vi "SQL查询.vi"(7 "condition":string, 8 "error in (no error)":errorcluster, 9 "columns":string[](array[string]), 10 "table输入":string(combo), 11 "database":string(combo)) -> (0 "error out":errorcluster, 1 "拆分数据":bool, 2 "columns输出":string[](array[string]), 3 "data":string[][](table))   [LabVIEW 2016, in "数据传输系统-02.lvlib"]
uses:
  <vilib>/Utility/sysdir.llb/System Directory Type.ctl
  <vilib>/addons/database/Connection.llb/DB Tools Open Connec (String).vi
  <vilib>/addons/database/_DB Variant To Data/Database Variant To Data.xnode
  <vilib>/addons/database/NI_Database_API.lvlib
panel:
  out "error out 2":errorcluster
  out "结果字符串":string
  out "元素":string
  out "子数组":string[](array[string])
  # "时间 > #2021/01/15 08:00:00#and 时间 < #2021/04/15 08:00:00# order by 时间 asc"
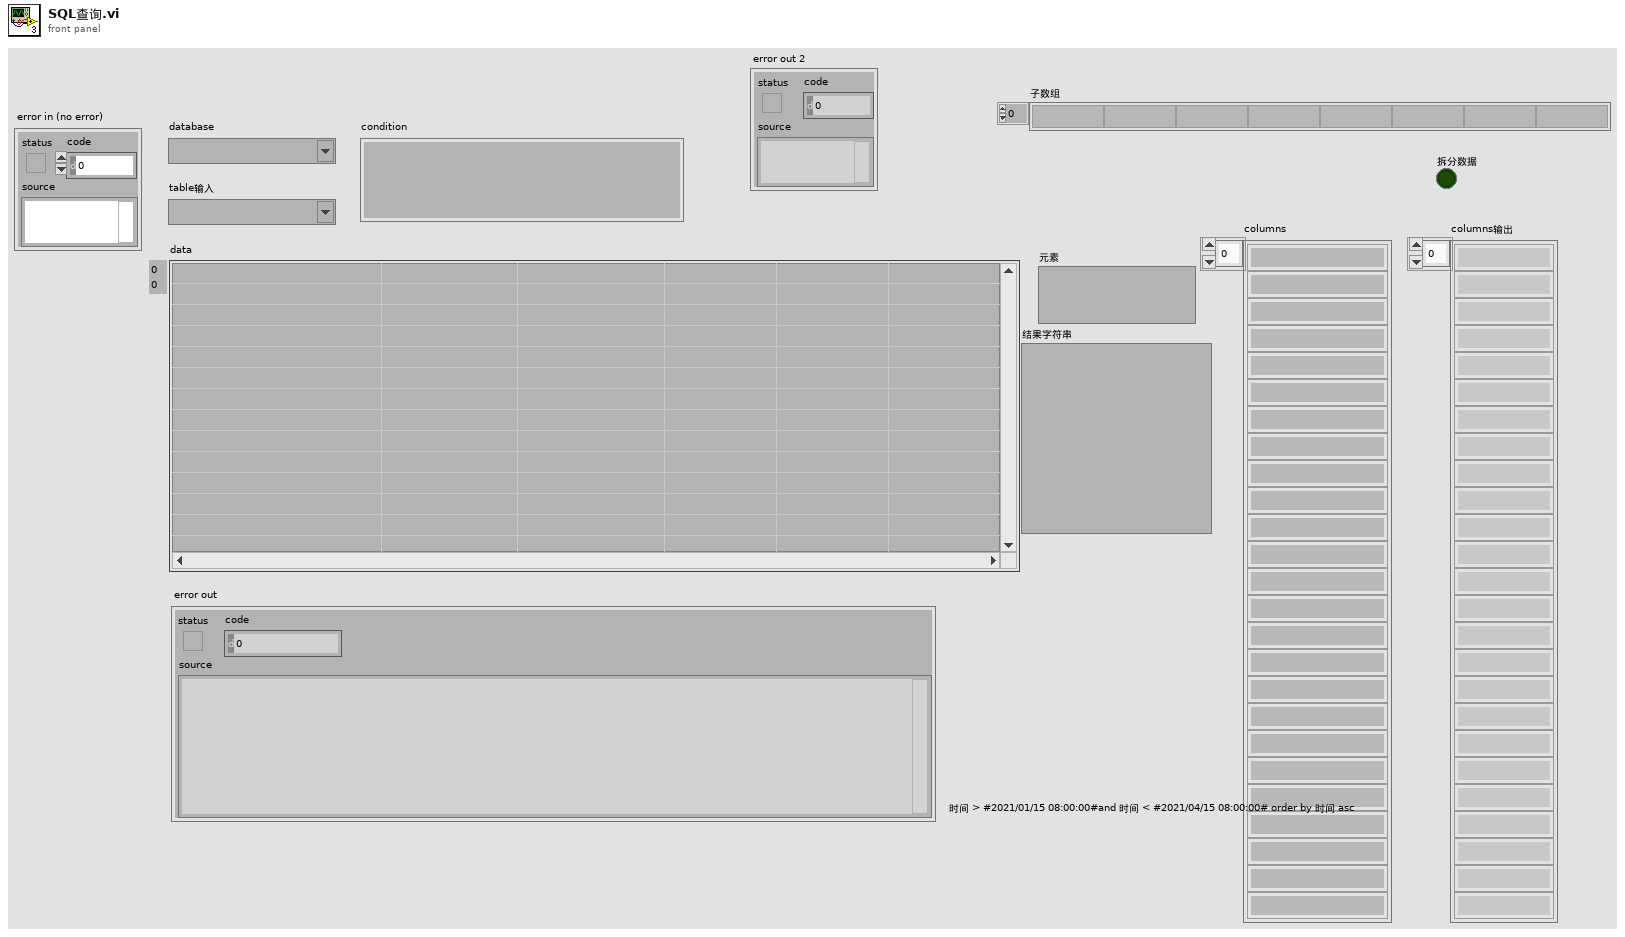
[diagram p1: front panel]
types:
  T1 = typedef "Semaphore RefNum" = refnum<k1>
  T2 = typedef "System Directory Type.ctl" = i32
  T3 = typedef "NI_Database_API.lvlib/Conn ObjectReference.ctl" = refnum<k1>
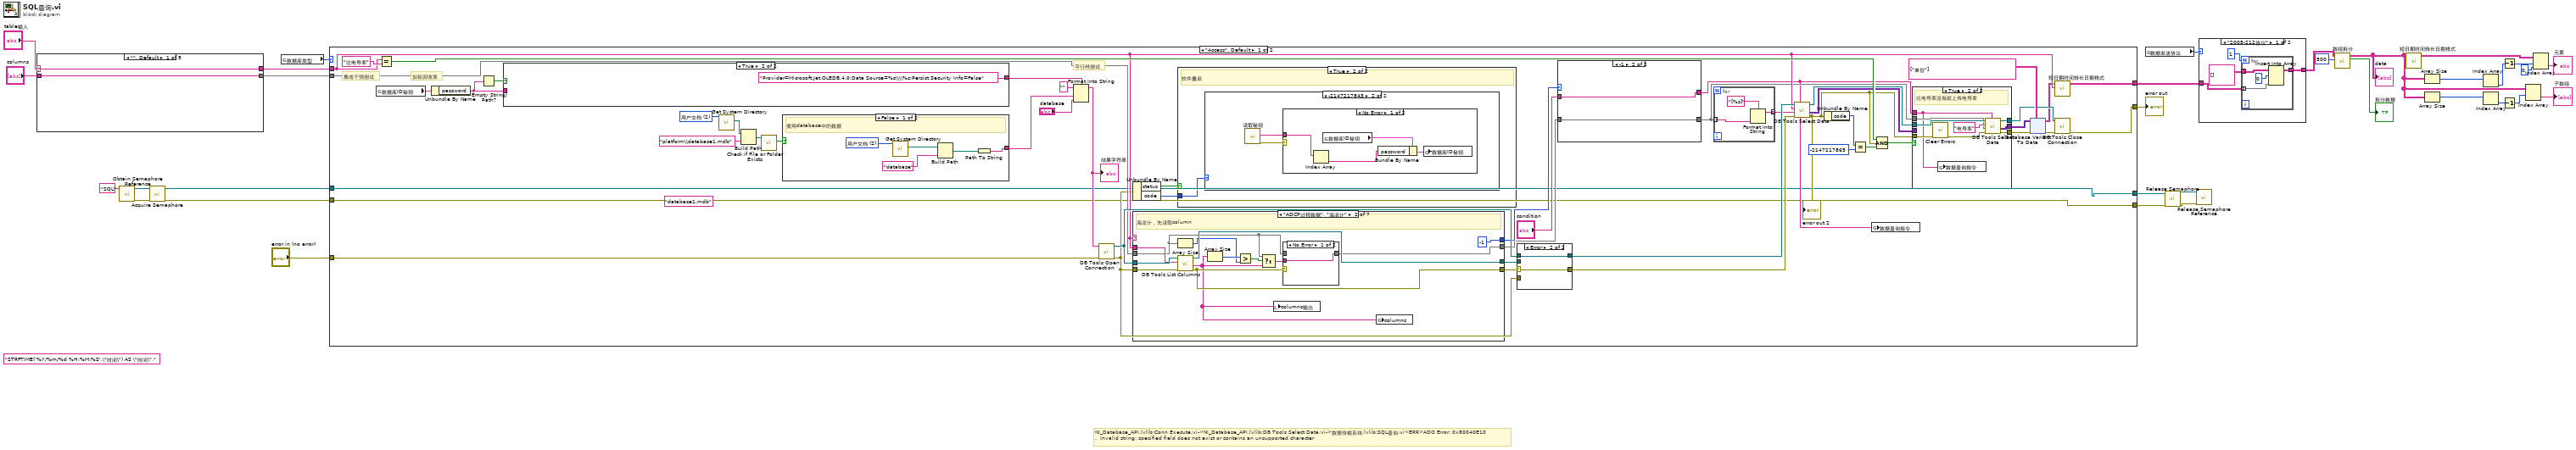
[diagram p0: block diagram]
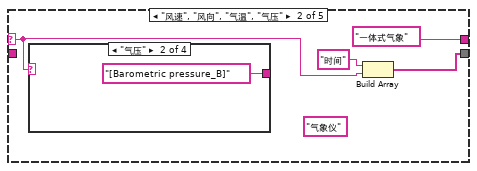
[diagram p2: hidden frame]
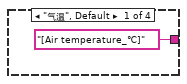
[diagram p3: hidden frame]
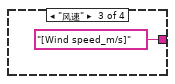
[diagram p4: hidden frame]
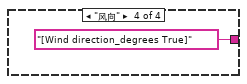
[diagram p5: hidden frame]
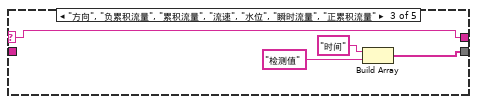
[diagram p6: hidden frame]
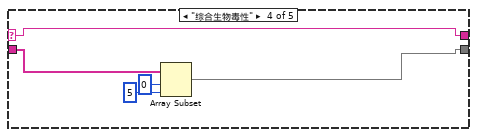
[diagram p7: hidden frame]
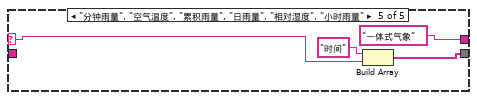
[diagram p8: hidden frame]
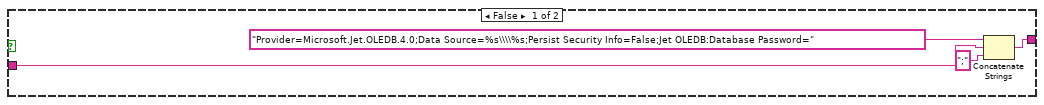
[diagram p9: hidden frame]
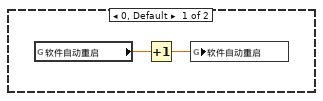
[diagram p11: hidden frame]
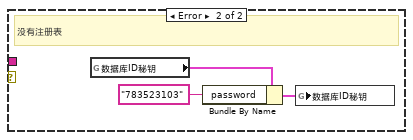
[diagram p12: hidden frame]
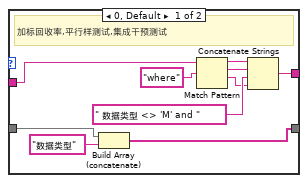
[diagram p13: hidden frame]
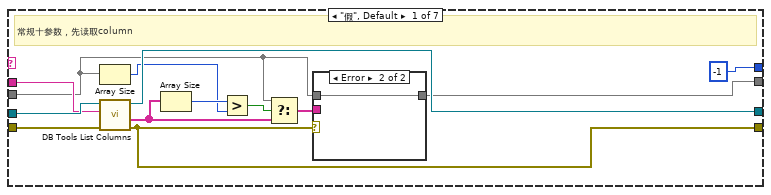
[diagram p15: hidden frame]
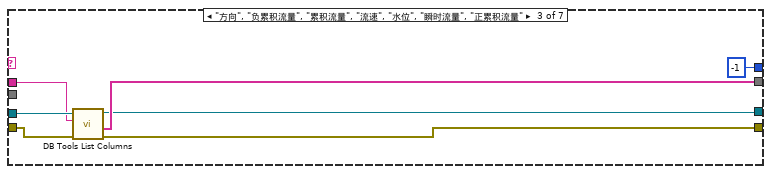
[diagram p18: hidden frame]
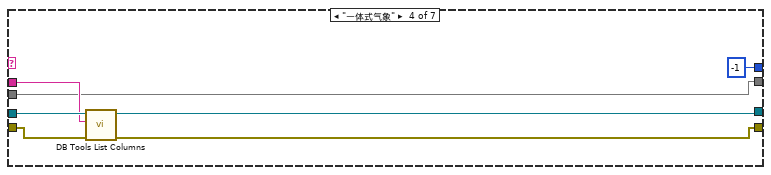
[diagram p19: hidden frame]
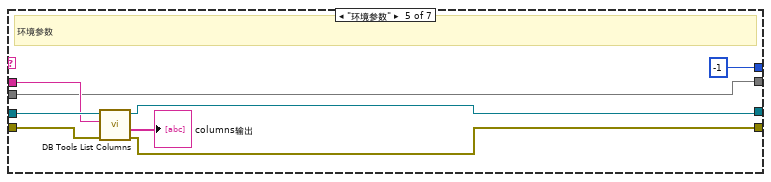
[diagram p20: hidden frame]
diagram:
  (unwired) "STRFTIME('%Y/%m/%d %H:%M:%S',\"时间\") AS \"时间\"," ("输入 1")
  # "NI_Database_API.lvlib:Conn Execute.vi->NI_Database_API.lvlib:DB Tools Select Data.vi->数据传输系统.lvlib:SQL查询.vi<ERR>ADO Error: 0x80040E10\n.  Invalid string: specified field does not exist or contains an unsupported character"
  n1 = case shown="\"\", Default" "table输入" {
    selector: "table输入" -> [w34 w36 w43 w51 w53]
    tunnel: [w34 "一体式气象" w43 w51 "一体式气象"] -> w13
    tunnel: "columns" -> [w33 _ _ w50 _]
    tunnel: [w33 w37 w45 w47 w54] -> w14
    frame "", Default {
    }
    frame "风速", "风向", "气温", "气压" {
      (unwired) "气象仪"
      n2 = case shown="\"气压\"" w36 {
        tunnel: ["[Air temperature_℃]" "[Barometric pressure_B]" "[Wind speed_m/s]" "[Wind direction_degrees True]"] -> _
        frame "气温", Default {
        }
        frame "气压" {
        }
        frame "风速" {
        }
        frame "风向" {
        }
      }
      n3 = Build Array("时间", w36) -> (w37:string[])
    }
    frame "方向", "负累积流量", "累积流量", "流速", "水位", "瞬时流量", "正累积流量" {
      n4 = Build Array("时间", "检测值") -> (w45:string[])
    }
    frame "综合生物毒性" {
      n5 = Array Subset(array=w50, index=0 ("索引"), length=5 ("长度")) -> (w47:string[])
    }
    frame "分钟雨量", "空气温度", "累积雨量", "日雨量", "相对湿度", "小时雨量" {
      n6 = Build Array("时间", w53) -> (w54:string[])
    }
  }
  n7 = call <vilib>:"Obtain Semaphore Reference.vi"("name (unnamed)"="SQL") -> ("error out"=w8:errorcluster, "semaphore"=w7:T1)  [unwired: 4 in, 1 out]
  n8 = call <vilib>:"Acquire Semaphore.vi"("error in (no error)"=w8, "semaphore"=w7) -> ("error out"=w5:errorcluster, "semaphore out"=w6:T1)  [unwired: 3 in, 1 out]
  n9 = global read "断电保存全局.vi" "数据库类型"() -> (w17:enum16{"Access", "SQLite"})
  n10 = case shown="\"Access\", Default" w17 {
    tunnel: [w101 w324] -> w32
    tunnel: [w77 w300] -> w20
    tunnel: "error in (no error)" -> [w72 w293]
    tunnel: w14 -> [w70 w296]
    tunnel: w13 -> [w69 w295]
    tunnel: w6 -> [w57 w290]
    tunnel: w5 -> [w56 w289]
    tunnel: [w57 w290] -> w4
    tunnel: [w56 w289] -> w3
    frame "Access", Default {
      (unwired) "database1.mdb" ("condition")
      w99 = T2 2 items=["用户目录"=0, "用户桌面"=1, "用户文档"=2, "用户应用程序数据"=3, "用户设置"=4, "用户临时目录"=5, "公共文档"=6, "公共应用程序数据"=7, "公共设置"=8, "公共缓存"=13, "系统核心库"=9, "系统安装库"=10, "应用程序文件"=11, "启动盘根目录"=12] ("system directory type")
      # "集成干预测试"
      # "平行样测试"
      # "加标回收率"
      n11 = global read "外部交互全局.vi" "数据库ID秘钥"() -> (w73:cluster{"userID":string, "password":string})
      n12 = Equal?(x=w69, y="比电导率") -> (x = y?=w95:bool)
      n13 = Unbundle By Name(w73) -> ("password"=w74:string)
      n14 = Empty String/Path?(string/path=w74) -> (empty?=w61:bool)
      n15 = case shown="True" w61 {
        tunnel: [w109 "Provider=Microsoft.Jet.OLEDB.4.0;Data Source=%s\\\\%s;Persist Security Info=False" ("格式字符串")] -> w75
        tunnel: w74 -> [w108 _]
        frame False {
          n16 = Concatenate Strings("Provider=Microsoft.Jet.OLEDB.4.0;Data Source=%s\\\\%s;Persist Security Info=False;Jet OLEDB:Database Password=" ("格式字符串"), w108, ";" ("字符串")) -> (w109:string)
        }
        frame True {
        }
      }
      n17 = call <vilib>:"Get System Directory.vi"("system directory type"=w99) -> ("system directory"=w100:path)  [unwired: 10 in]
      n18 = Build Path(base path=w100, name or relative path="platform\\database1.mdb" ("condition")) -> (appended path=w98:path)
      n19 = call <vilib>:"Check if File or Folder Exists.vi"("path"=w98) -> ("file or folder exists?"=w58:bool)  [unwired: 8 in, 2 out]
      n20 = case shown="False" w58 {
        tunnel: [w235 w240] -> w97
        frame False {
          w238 = T2 2 items=["用户目录"=0, "用户桌面"=1, "用户文档"=2, "用户应用程序数据"=3, "用户设置"=4, "用户临时目录"=5, "公共文档"=6, "公共应用程序数据"=7, "公共设置"=8, "公共缓存"=13, "系统核心库"=9, "系统安装库"=10, "应用程序文件"=11, "启动盘根目录"=12] ("system directory type")
          # "使用database中的数据"
          n21 = call <vilib>:"Get System Directory.vi"("system directory type"=w238) -> ("system directory"=w237:path)  [unwired: 10 in]
          n22 = Build Path(base path=w237, name or relative path="database" ("condition")) -> (appended path=w239:path)
          n23 = Path To String(path=w239) -> (string=w235:string)
        }
        frame True {
          w244 = T2 2 items=["用户目录"=0, "用户桌面"=1, "用户文档"=2, "用户应用程序数据"=3, "用户设置"=4, "用户临时目录"=5, "公共文档"=6, "公共应用程序数据"=7, "公共设置"=8, "公共缓存"=13, "系统核心库"=9, "系统安装库"=10, "应用程序文件"=11, "启动盘根目录"=12] ("system directory type")
          # "使用platform中的数据"
          n24 = call <vilib>:"Get System Directory.vi"("system directory type"=w244) -> ("system directory"=w243:path)  [unwired: 10 in]
          n25 = Build Path(base path=w243, name or relative path="platform" ("condition")) -> (appended path=w241:path)
          n26 = Path To String(path=w241) -> (string=w240:string)
        }
      }
      n27 = Format Into String(format string=w75, initial string="" ("初始字符串"), w97, "database") -> (resulting string=w65:string)  [unwired: 1 in, 1 out]
      "结果字符串" <- w65
      n28 = call-poly <vilib>:"DB Tools Open Connection.vi"("error in (no error)"=w72, "connection information"=w65) -> ("error out"=w62:errorcluster, "connection reference"=w81:T3)  [unwired: 6 in]
      n29 = Unbundle By Name(w62) -> ("status"=w76:bool, "code"=w68:i32)
      n30 = case shown="\"ADCP过程数据\", \"海流计\"" w69 {
        tunnel: w81 -> [w152 w167 w177 w184 w192 w200 w222]
        tunnel: w62 -> [w149 w164 w175 w183 w191 w199 w220]
        tunnel: [w150 w165 w172 w181 w190 w197 w219] -> w83
        tunnel: [w144 w160 w171 w180 w189 w198 w218] -> w84
        tunnel: w69 -> [w151 w166 w176 w182 w188 w201 w221]
        tunnel: [-1 ("index of element") -1 ("index of element") -1 ("index of element") -1 ("index of element") -1 ("index of element") -1 ("index of element") w215] -> w79
        tunnel: w70 -> [w141 w157 _ w178 w185 w196 w214]
        tunnel: [w142 w158 w174 w178 w185 w193 w214] -> w78
        frame "假", Default {
          # "常规十参数，先读取column"
          n31 = Array Size(array=w141) -> (size(s)=w146:i32)
          n32 = call <vilib>:"DB Tools List Columns.vi"("error in (no error)"=w149, "table"=w151, "connection reference"=w152) -> ("error out"=w144:errorcluster, "columns"=w145:string[], "connection reference out"=w150:T3)  [unwired: 1 in, 1 out]
          n33 = Array Size(array=w145) -> (size(s)=w147:i32)
          n34 = Greater?(x=w147, y=w146) -> (0:w148:bool)
          n35 = Select(t=w141, s=w148, f=w145) -> (s? t:f=w143:string[])
          n36 = case shown="Error" w144 {
            tunnel: w143 -> [w154 _]
            tunnel: [w154 w155] -> w142
            tunnel: w141 -> [_ w155]
            frame No Error {
            }
            frame Error {
            }
          }
        }
        frame "ADCP过程数据", "海流计" {
          # "海流计，先读取column"
          n37 = Array Size(array=w157) -> (size(s)=w161:i32)
          n38 = call <vilib>:"DB Tools List Columns.vi"("error in (no error)"=w164, "table"=w166, "connection reference"=w167) -> ("error out"=w160:errorcluster, "columns"=w156:string[], "connection reference out"=w165:T3)  [unwired: 1 in, 1 out]
          n39 = Array Size(array=w156) -> (size(s)=w162:i32)
          n40 = Greater?(x=w162, y=w161) -> (0:w163:bool)
          n41 = Select(t=w157, s=w163, f=w156) -> (s? t:f=w159:string[])
          n42 = local write "columns输出"(w156) -> ()
          n43 = case shown="No Error" w160 {
            tunnel: w159 -> [w169 _]
            tunnel: [w169 w170] -> w158
            tunnel: w157 -> [_ w170]
            frame No Error {
            }
            frame Error {
            }
          }
          n44 = global write "全局 所有参数.vi" "columns"(w156) -> ()
        }
        frame "方向", "负累积流量", "累积流量", "流速", "水位", "瞬时流量", "正累积流量" {
          n45 = call <vilib>:"DB Tools List Columns.vi"("error in (no error)"=w175, "table"=w176, "connection reference"=w177) -> ("error out"=w171:errorcluster, "columns"=w174:string[], "connection reference out"=w172:T3)  [unwired: 1 in, 1 out]
        }
        frame "一体式气象" {
          n46 = call <vilib>:"DB Tools List Columns.vi"("error in (no error)"=w183, "table"=w182, "connection reference"=w184) -> ("error out"=w180:errorcluster, "connection reference out"=w181:T3)  [unwired: 1 in, 2 out]
        }
        frame "环境参数" {
          # "环境参数"
          n47 = call <vilib>:"DB Tools List Columns.vi"("error in (no error)"=w191, "table"=w188, "connection reference"=w192) -> ("error out"=w189:errorcluster, "columns"=→"columns输出":string[], "connection reference out"=w190:T3)  [unwired: 1 in, 1 out]
        }
        frame "剖面数据" {
          # "环境参数"
          n48 = call <vilib>:"DB Tools List Columns.vi"("error in (no error)"=w199, "table"=w201, "connection reference"=w200) -> ("error out"=w198:errorcluster, "columns"=w195:string[], "connection reference out"=w197:T3)  [unwired: 1 in, 1 out]
          n49 = for {
            tunnel: w196 -> [w205] mode=indexing
            tunnel: w195 -> [w209]
            shift-right: [w203] -> w193
            shift-left: string[] [] -> [w206]
            n50 = Search 1D Array(1D array=w209, element=w205) -> (index of element=w208:i32)  [unwired: 1 in]
            n51 = Not Equal?(x=w208, y=-1) -> (x != y?=w204:bool)
            n52 = case shown="True" w204 {
              tunnel: w206 -> [w210 w213]
              tunnel: w205 -> [_ w212]
              tunnel: [w210 w211] -> w203
              frame False {
              }
              frame True {
                n53 = Build Array (concatenate)(w213, w212) -> (w211:string[])
              }
            }
          }
          n54 = local write "columns输出"(w193) -> ()
        }
        frame "集成干预测试", "加标回收率", "平行样测试" {
          n55 = call <vilib>:"DB Tools List Columns.vi"("error in (no error)"=w220, "table"=w221, "connection reference"=w222) -> ("error out"=w218:errorcluster, "columns"=w217:string[], "connection reference out"=w219:T3)  [unwired: 1 in, 1 out]
          n56 = Search 1D Array(1D array=w217, element="数据类型" ("元素")) -> (index of element=w215:i32)  [unwired: 1 in]
        }
      }
      n57 = case shown="True" w76 {
        tunnel: w68 -> [_ w113]
        frame False {
        }
        frame True {
          # "软件重启"
          n58 = case shown="-2147217843" w113 {
            frame 0, Default {
              n59 = global read "全局1.vi" "软件自动重启"() -> (w115:dbl)
              n60 = Increment(x=w115) -> (x+1=w114:dbl)
              n61 = global write "全局1.vi" "软件自动重启"(w114) -> ()
            }
            frame -2147217843 {
              n62 = call "读取秘钥.vi"() -> ("error out"=w116:errorcluster, "值"=w117:string[])  [unwired: 9 in, 1 out]
              n63 = case shown="No Error" w116 {
                tunnel: w117 -> [w121 _]
                frame No Error {
                  n64 = Index Array(array=w121) -> (element=w118:string)  [unwired: 1 in]
                  n65 = global read "外部交互全局.vi" "数据库ID秘钥"() -> (w119:cluster{"userID":string, "password":string})
                  n66 = Bundle By Name(cluster=w119, "password"=w118) -> (w120:cluster{"userID":string, "password":string})
                  n67 = global write "外部交互全局.vi" "数据库ID秘钥"(w120) -> ()
                }
                frame Error {
                  # "没有注册表"
                  n68 = global read "外部交互全局.vi" "数据库ID秘钥"() -> (w123:cluster{"userID":string, "password":string})
                  n69 = Bundle By Name(cluster=w123, "password"="783523103") -> (w124:cluster{"userID":string, "password":string})
                  n70 = global write "外部交互全局.vi" "数据库ID秘钥"(w124) -> ()
                }
              }
            }
          }
        }
      }
      n71 = case shown="Error" w84 {
        selector: w84 -> [_ w140]
        tunnel: w83 -> [w138 _]
        tunnel: [w138 w139] -> w82
        tunnel: w81 -> [_ w139]
        tunnel: [w137 w140] -> w80
        tunnel: w62 -> [w137 _]
        frame No Error {
        }
        frame Error {
        }
      }
      n72 = case "条件结构" shown="-1" w79 {
        tunnel: "condition" -> [w132 w135]
        tunnel: w78 -> [w134 w136]
        tunnel: [w126 w136] -> w67
        tunnel: [w125 w135] -> w60
        frame 0, Default {
          # "加标回收率,平行样测试,集成干预测试"
          n73 = Build Array (concatenate)(w134, "数据类型" ("元素")) -> (w126:string[])
          n74 = Match Pattern(string=w132, regular expression="where" ("正则表达式")) -> (before substring=w130:string, match substring=w129:string, after substring=w127:string)  [unwired: 1 in, 1 out]
          n75 = Concatenate Strings(w130, w129, " 数据类型 <> 'M' and " ("字符串"), w127) -> (w125:string)
        }
        frame -1 {
        }
      }
      n76 = for {
        tunnel: w67 -> [w107] mode=indexing
        tunnel: [w106] -> w66 mode=indexing
        n77 = Format Into String(format string="[%s]" ("格式字符串"), w107) -> (resulting string=w106:string)  [unwired: 2 in, 1 out]
      }
      n78 = call <vilib>:"DB Tools Select Data.vi"("condition"=w60, "error in (no error)"=w80, "columns"=w66, "table"=w69, "connection reference"=w82) -> ("error out"=w88:errorcluster, "data"=w90:variant[][], "connection reference out"=w93:T3)  [unwired: 1 in]
      "error out 2" <- w88
      n79 = Unbundle By Name(w88) -> ("code"=w87:i32)
      n80 = Equal?(x=w87, y=-2147217865 ("code")) -> (x = y?=w85:bool)
      n81 = global write "全局 水样时间.vi" "数据查询指令"(w60) -> ()
      n82 = Compound Arithmetic op=AND ("复合运算")(w95, w88, w85) -> (w94:bool)
      n83 = case shown="True" w94 {
        tunnel: w60 -> [_ w226]
        tunnel: w93 -> [w225 w234]
        tunnel: [w225 w229] -> w92
        tunnel: [w224 w230] -> w91
        tunnel: w90 -> [w224 _]
        tunnel: w88 -> [w223 w232]
        tunnel: [w223 w228] -> w89
        tunnel: w67 -> [_ w227]
        frame False {
        }
        frame True {
          # "比电导率没有就上传电导率"
          n84 = call <vilib>:"Clear Errors.vi"("error in (no error)"=w232) -> ("error out"=w231:errorcluster)  [unwired: 5 in, 1 out]
          n85 = global write "全局 水样时间.vi" "数据查询指令"(w226) -> ()
          n86 = call <vilib>:"DB Tools Select Data.vi"("condition"=w226, "error in (no error)"=w231, "columns"=w227, "table"="电导率", "connection reference"=w234) -> ("error out"=w228:errorcluster, "data"=w230:variant[][], "connection reference out"=w229:T3)  [unwired: 1 in]
        }
      }
      n87 = xnode "Database Variant To Data"("database variant"=w91, "error in (no error)"=w89, "type"=string[][] [["单位"]]) -> ("data"=w64:string[][], "error out"=w102:errorcluster)
      n88 = call "短日期时间转长日期格式.vi"("table输入"=w69, "data"=w64) -> ("输出数组"=w101:string[][])  [unwired: 9 in]
      n89 = call <vilib>:"DB Tools Close Connection.vi"("error in (no error)"=w102, "connection reference"=w92) -> ("error out"=w77:errorcluster)  [unwired: 5 in]
    }
    frame "SQLite" {
      w298 = "比电导率" ("y")
      (unwired) "order by STRFTIME('%Y/%m/%d %H:%M:%S',\"时间\")" ("替换字符串(\"\")")
      (unwired) "order by 时间" ("搜索字符串")
      w309 = TRUE ("替换全部？(F)")
      w326 = T2 2 items=["用户目录"=0, "用户桌面"=1, "用户文档"=2, "用户应用程序数据"=3, "用户设置"=4, "用户临时目录"=5, "公共文档"=6, "公共应用程序数据"=7, "公共设置"=8, "公共缓存"=13, "系统核心库"=9, "系统安装库"=10, "应用程序文件"=11, "启动盘根目录"=12] ("system directory type")
      n90 = local write "columns输出"(w296) -> ()
      n91 = local read "condition"() -> (w308:string)
      n92 = case shown="\"假\", Default" w295 {
        tunnel: w308 -> [w340 w346]
        tunnel: w296 -> [w339 w348]
        tunnel: [w339 w347] -> w319
        tunnel: [w340 w345] -> w307
        frame "假", Default {
        }
        frame "集成干预测试", "加标回收率", "平行样测试" {
          n93 = Build Array (concatenate)(w348, "数据类型" ("元素")) -> (w347:string[])
          n94 = call "数据库加密匹配 (子VI).vi"("输入参数"="N") -> ("Encoded String"=w343:string)  [unwired: 10 in]
          n95 = Match Pattern(string=w346, regular expression="where" ("正则表达式")) -> (before substring=w351:string, match substring=w350:string, after substring=w349:string)  [unwired: 1 in, 1 out]
          n96 = Format Into String(format string=" 数据类型 = '%s' and " ("字符串"), w343) -> (resulting string=w341:string)  [unwired: 2 in, 1 out]
          n97 = Concatenate Strings(w351, w350, w341, w349) -> (w345:string)
        }
      }
      n98 = local read "database"() -> (w311:string)
      n99 = Array Size(array=w319) -> (size(s)=w323:i32)
      n100 = call <vilib>:"Get System Directory.vi"("system directory type"=w326) -> ("system directory"=w325:path)  [unwired: 10 in]
      n101 = Search and Replace String(replace all?=w309, input string=w307, search string="/" ("搜索字符串"), replace string="-" ("替换字符串(\"\")")) -> (result string=w316:string)  [unwired: 4 in, 3 out]
      n102 = Equal To 0?(x=w323) -> (x = 0?=w322:bool)
      n103 = Build Path(base path=w325, name or relative path="Platform\\database1.db" ("condition")) -> (appended path=w327:path)
      n104 = case shown="False" w322 {
        tunnel: w319 -> [_ w356]
        tunnel: ["*" ("t") w355] -> w320
        frame True {
        }
        frame False {
          n105 = call <userlib>:"SQLite_Implode 1D.vi"("Values"=w356, "format string"="%s") -> ("imploded string"=w355:string)  [unwired: 7 in, 1 out]
        }
      }
      n106 = call <vilib>:"Check if File or Folder Exists.vi"("path"=w327) -> ("file or folder exists?"=w329:bool)  [unwired: 8 in, 2 out]
      n107 = Search and Replace String(replace all?=TRUE ("替换全部？(F)"), input string=w311, search string=".mdb" ("搜索字符串"), replace string=".db" ("替换字符串(\"\")")) -> (result string=w306:string)  [unwired: 4 in, 3 out]
      n108 = Search and Replace String(replace all?=w309, input string=w316, search string="#" ("搜索字符串"), replace string="'" ("替换字符串(\"\")")) -> (result string=w291:string)  [unwired: 4 in, 3 out]
      n109 = case shown="False" w329 {
        tunnel: [w359 w360] -> w294
        tunnel: w306 -> [w358 w361]
        frame False {
          # "使用database中的数据"
          n110 = call "database path.vi"("database"=w358) -> ("Path out"=w359:string)  [unwired: 9 in, 1 out]
        }
        frame True {
          # "使用platform中的数据"
          n111 = call "database platform path.vi"("database"=w361) -> ("Path out"=w360:string)  [unwired: 10 in]
        }
      }
      n112 = Format Into String(format string="SELECT %s %s FROM `%s` %s;" ("SQL Query"), "", w320, w295, w291) -> (resulting string=w301:string)  [unwired: 2 in, 1 out]
      n113 = call "Sqlite Query.vi"("DB Path"=w294, "SQL Query"=w301, "error in (no error)"=w293) -> ("Results"=w303:string[][], "DB Path Out"=w297:string, "error out"=w299:errorcluster)  [unwired: 10 in]
      n114 = Equal?(x=w295, y=w298) -> (x = y?=w305:bool)
      n115 = And(x=w299, y=w305) -> (x .and. y?=w304:bool)
      n116 = case shown="True" w304 {
        tunnel: w303 -> [w331 _]
        tunnel: [w331 w338] -> w302
        tunnel: w301 -> [_ w335]
        tunnel: w297 -> [_ w337]
        tunnel: [w330 w336] -> w300
        tunnel: w299 -> [w330 _]
        tunnel: w298 -> [_ w334]
        frame False {
        }
        frame True {
          n117 = Search and Replace String(input string=w335, search string=w334, replace string="电导率" ("Tables Name")) -> (result string=w332:string)  [unwired: 5 in, 3 out]
          n118 = call "Sqlite Query.vi"("DB Path"=w337, "SQL Query"=w332) -> ("Results"=w338:string[][], "error out"=w336:errorcluster)  [unwired: 11 in, 1 out]
        }
      }
      n119 = call "短日期时间转长日期格式.vi"("data"=w302) -> ("输出数组"=w324:string[][])  [unwired: 10 in]
    }
  }
  "error out" <- w20
  n120 = global read "断电保存全局.vi" "数据发送协议"() -> (w31:enum16{"2005-212协议", "2017-212协议"})
  n121 = call <vilib>:"Release Semaphore.vi"("error in (no error)"=w3, "semaphore"=w4) -> ("error out"=w1:errorcluster, "semaphore out"=w2:T1)  [unwired: 4 in]
  n122 = call <vilib>:"Release Semaphore Reference.vi"("error in (no error)"=w1, "semaphore"=w2) -> ()  [unwired: 8 in, 2 out]
  n123 = case shown="\"2005-212协议\"" w31 {
    tunnel: w32 -> [w363 w370]
    tunnel: [w362 w370] -> w18
    frame "2005-212协议" {
      n124 = for {
        N: 1 -> [_]
        tunnel: string[][] [] ("data") -> [w369]
        tunnel: w363 -> [w368] mode=indexing
        tunnel: [w366] -> w362
        n125 = Insert Into Array(array=w369, index (row)=0 ("索引 (行)"), new element=w368) -> (w366:string[][])  [unwired: 1 in]
      }
    }
    frame "2017-212协议", Default {
    }
  }
  n126 = call "数组拆分.vi"("拆分大小"=500, "输入数据"=w18) -> ("拆分数据"=→"拆分数据":bool, "输出数组"=w10:string[][])  [unwired: 8 in]
  "data" <- w10
  n127 = call "短日期时间转长日期格式.vi"("data"=w10) -> ("输出数组"=w26:string[][])  [unwired: 10 in]
  n128 = Array Size(array=w10) -> (size(s)=w25:i32[])
  n129 = Array Size(array=w10) -> (size(s)=w30:i32[])
  n130 = Index Array(array=w25) -> (element=w24:i32)  [unwired: 1 in]
  n131 = Index Array(array=w30) -> (element=w28:i32)  [unwired: 1 in]
  n132 = Decrement(x=w24) -> (x-1=w23:i32)
  n133 = Decrement(x=w28) -> (x-1=w27:i32)
  n134 = Index Array(array=w10, index (row)=w27) -> (element=→"子数组":string[])  [unwired: 1 in]
  n135 = Index Array(array=w26, index (row)=w23, index (col)=0 ("禁用的索引 (列)")) -> (element=→"元素":string)
